vi "500 Hz Cut Off.vi"() -> ()   [LabVIEW 2016]
uses:
  <vilib>/rvi/Emulation/niFpgaGetClockAttributes.vi
  <vilib>/rvi/Emulation/niFpgaSctlEmulationGetInTimedLoop.vi
  <vilib>/rvi/Emulation/niFpgaEmulationReportErrorSimple.vi
  <vilib>/rvi/eio/common/nirviEmuTemplateMethod_errors.vi
  <vilib>/rvi/Emulation/niFpgaCriticalErrorInLSC.vi
  <vilib>/eio/EIONode/EIONode.xnode
  <vilib>/rvi/Analysis/measure/butterworth/XNode/niFpgaButterworthFilter.xnode
panel:
  in  "DIO0":bool=TRUE
  out "Boolean":bool
  out "Unfiltered Signal":sgl
  out "Filtered Signal":fxp<+/-,28,9>
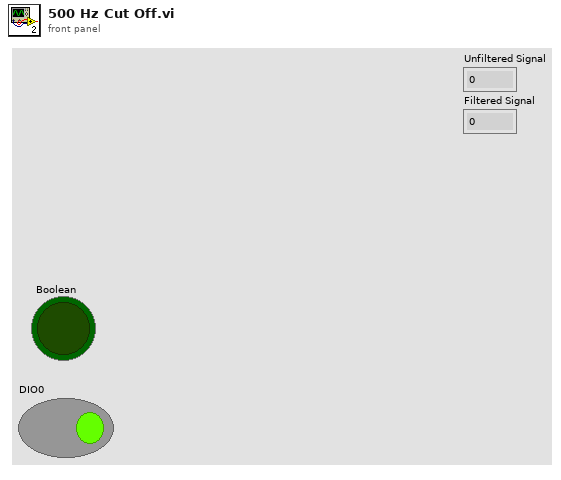
[diagram p1: front panel]
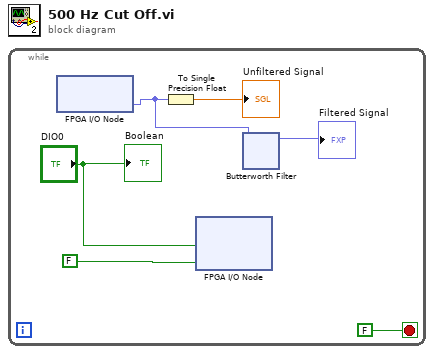
[diagram p0: block diagram]
diagram:
  n1 = while {
    stop <- FALSE ("stop") stop-if-true
    n2 = xnode "FPGA I/O Node"() -> ("AI0"=w2:fxp<+/-,24,5>)  [unwired: 1 in, 1 out]
    n3 = To Single Precision Float(number=w2) -> (single precision float=→"Unfiltered Signal":sgl)
    n4 = xnode "FPGA I/O Node"("DIO0"="DIO0", "DIO3"=FALSE) -> ()  [unwired: 2 in, 2 out]
    n5 = xnode "Butterworth Filter"("input data"=w2) -> ("output data"=→"Filtered Signal":fxp<+/-,24,5>)  [unwired: 2 in]
    "Boolean" <- "DIO0"
  }
